vi "Begin.vi"(8 "error in":errorcluster) -> (0 "error out":errorcluster)   [LabVIEW 2017]
doc: "Called before other user functions, this VI is expected to open initial I/O refnums, load in file data, and do all program initialization. Notice that the <B>error out</B> terminal is simply used for data flow. Wiring it to other structures or subVIs ensures that this VI runs first."
uses:
  <vilib>/Rock Robotics/WPI/DriverStation/WPI_DriverStationRobotMode2.ctl
  <vilib>/Rock Robotics/WPI/Joystick/WPI_JoystickDeviceEnum.ctl
  <vilib>/Rock Robotics/WPI/SafetyOutput/WPI_SafetyOutputConfigMenu.ctl
  <vilib>/Rock Robotics/WPI/ThirdParty/Phoenix-LabVIEW/Motor Controller/Controls/CTRE_Phoenix_MotorControl_FeedbackDevice.ctl
  <vilib>/Rock Robotics/WPI/Solenoid/WPI_SolenoidChannel.ctl
  Robot Global Data.vi
  <vilib>/Rock Robotics/Network Tables/NT Write String Array.vi
  <vilib>/Rock Robotics/WPI/Utilities/WPI_GetSetVariantRefNum.vi
  <vilib>/Rock Robotics/WPI/RobotDrive/WPI_RobotDriveOpen4MotorWithExistingMotors.vi
  <vilib>/Rock Robotics/WPI/Solenoid/WPI_SolenoidOpenDouble.vi
  <vilib>/Rock Robotics/WPI/Solenoid/WPI_SolenoidOpenSingle.vi
  <vilib>/Rock Robotics/SystemInterfaces/spilib/spi_bus.ctl
  <vilib>/Rock Robotics/WPI/Gyro/WPI_GyroXRS450_SPI_Open.vi
  navx-mxp/labview/navX Library v2/navX Library v2.lvlib
  navx-mxp/labview/navX Library v2/IO/Open/Z900_navX_Open_I2C.vi
  <vilib>/Rock Robotics/SystemInterfaces/i2clib/i2c_bus.ctl
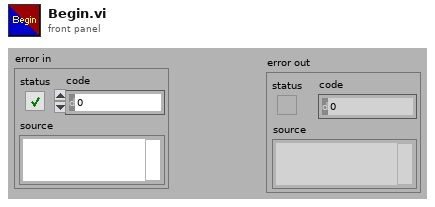
[diagram p1: front panel]
types:
  T1 = typedef "CTRE_Phoenix_MotorControl_FeedbackDevice.ctl" = i8
  T2 = typedef "WPI_JoystickDeviceEnum.ctl" = enum16{"USB 0", "USB 1", "USB 2", "USB 3", "USB 4", "USB 5"}
  T3 = typedef "WPI_SafetyOutputConfigMenu.ctl" = enum16{"Enable", "Disable"}
  T4 = typedef "WPI_DriverStationRobotMode2.ctl" = enum16{"Autonomous Disabled", "Autonomous Enabled", "Teleop Disabled", "Teleop Enabled", "Disconnected", "Finish", "Test Disabled", "Test Enabled", "Emergency Stopped"}
  T5 = typedef "WPI_MotorControlDeviceRef.ctl" = cluster{"DeviceStatus":errorcluster, "Type":T6, "PWM":cluster{"PWM Channel":T7, "DeadBand":T8}, "CAN":cluster{"Device Number":u8, "SetOutput VI Ref":variant, "GetOutput VI Ref":variant, "Enable VI Ref":variant, "Disable VI Ref":variant, "Data":variant}, "Invert":bool, "DIO PWM":cluster{"PWM \"Enable\" Channel":T7, "DIOChannel":T9, "PWM Rate":dbl}}
  T6 = typedef "WPI_MotorControlType.ctl" = enum16{"PWM", "CAN", "DIO PWM"}
  T7 = typedef "FPGA_DIOPWMChannel.ctl" = enum8{"PWM 0", "PWM 1", "PWM 2", "PWM 3", "PWM 4", "PWM 5", "PWM 6", "PWM 7", "PWM 8", "PWM 9", "PWM MXP 0", "PWM MXP 1", "PWM MXP 2", "PWM MXP 3", "PWM MXP 4", "PWM MXP 5", "PWM MXP 6", "PWM MXP 7", "PWM MXP 8", "PWM MXP 9", "Invalid"}
  T8 = typedef "WPI_PWMDeadband.ctl" = cluster{"Name":string, "maxPositivePwm":i32, "minPositivePwm":i32, "centerPwm":i32, "maxNegativePwm":i32, "minNegativePwm":i32, "angularRange":u16}
  T9 = typedef "FPGA_DIOChannel.ctl" = enum8{"DIO 0", "DIO 1", "DIO 2", "DIO 3", "DIO 4", "DIO 5", "DIO 6", "DIO 7", "DIO 8", "DIO 9", "DIO MXP 0", "DIO MXP 1", "DIO MXP 2", "DIO MXP 3", "DIO MXP 4", "DIO MXP 5", "DIO MXP 6", "DIO MXP 7", "DIO MXP 8", "DIO MXP 9", "DIO MXP 10", "DIO MXP 11", "DIO MXP 12", "DIO MXP 13", "DIO MXP 14", "DIO MXP 15", "SPI Port CS1", "SPI Port CS2", "SPI Port CS3", "SPI Port MISO", "SPI Port MOSI", "Invalid"}
  T10 = typedef "WPI_RobotDriveDevRef.ctl" = cluster{"DevStatus":errorcluster, "Motors[]":T5[], "Square Inputs":bool, "Max Output":dbl}
  T11 = typedef "i2c_bus.ctl" = enum16{"I2C On-Board", "I2C MXP", "Invalid"}
  T12 = typedef "navX Library v2.lvlib/Z900_navX_DeviceTypeDef.ctl" = cluster{"Interface":cluster{"Protocol":T13, "Update Rate (4Hz-100Hz)":u8, "navX Open TypeDef":variant}, "Notify Packet":refnum<notifier>, "Loop VI Refnum":refnum<vi>, "Ready to Close Occurrence Refnum":refnum<k4>}
  T13 = typedef "navX Library v2.lvlib/Z900_navX_ProtocolTypeDef.ctl" = enum16{"SERIAL", "I2C", "SPI"}
  T14 = typedef "spi_bus.ctl" = enum16{"SPI On-Board, CS0", "SPI On-Board, CS1", "SPI On-Board, CS2", "SPI On-Board, CS3", "SPI MXP", "Invalid"}
  T15 = typedef "WPI_GyroDevRef.ctl" = cluster{"DevStatus":errorcluster, "Analog Channel":T16, "Gain (VoltsPerDegree/Second)":dbl, "Gyro Type":enum16{"Analog", "XRS450"}, "Handle":i32, "SPI Bus":T14, "Device Found":bool, "Sample Rate":dbl, "Calibrate On Open":bool, "Offset":dbl}
  T16 = typedef "FPGA_AIChannel.ctl" = enum8{"AI 0", "AI 1", "AI 2", "AI 3", "AI MXP 0", "AI MXP 1", "AI MXP 2", "AI MXP 3", "Invalid"}
  T17 = typedef "WPI_SolenoidChannel.ctl" = enum8{"Solenoid 0", "Solenoid 1", "Solenoid 2", "Solenoid 3", "Solenoid 4", "Solenoid 5", "Solenoid 6", "Solenoid 7", "Invalid"}
  T18 = typedef "WPI_SolenoidDevRef.ctl" = cluster{"DevStatus":errorcluster, "Pneumatics Control Module":u8, "Forward Solenoid Channel":T17, "Reverse Solenoid Channel":T17}
  T19 = typedef "WPI_CompressorDevRef.ctl" = cluster{"DevStatus":errorcluster, "Pneumatics Control Module":u8}
  T20 = typedef "WPI_JoystickDevRef.ctl" = cluster{"Device":T2}
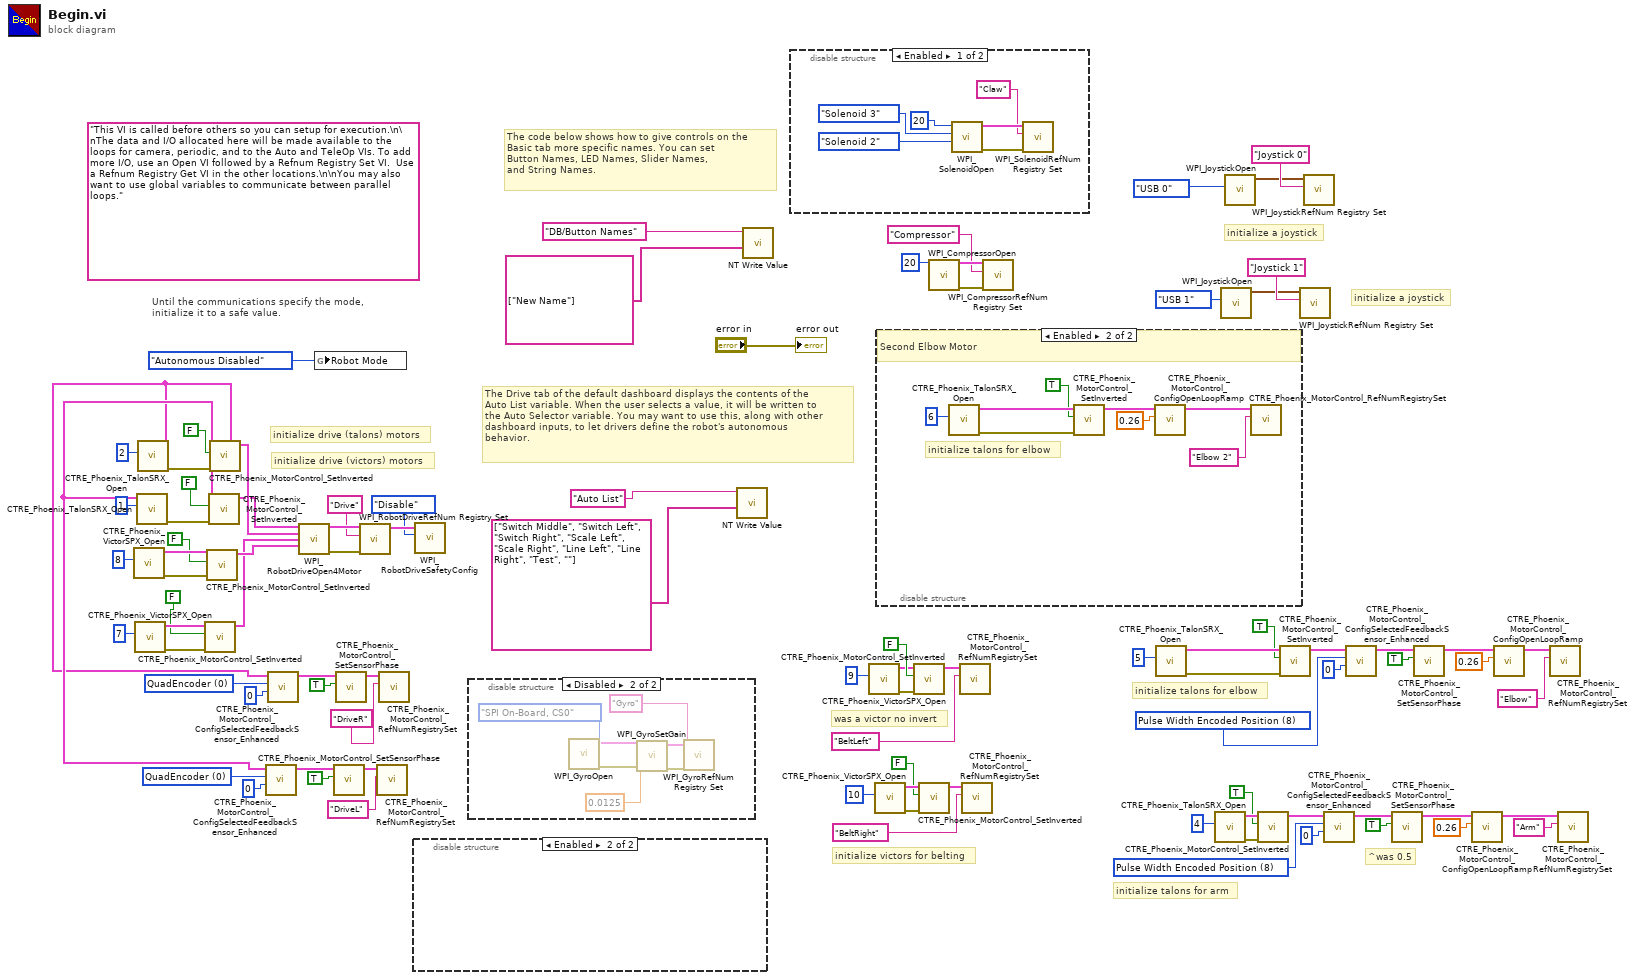
[diagram p0: block diagram]
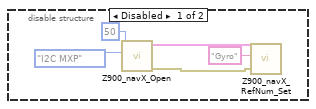
[diagram p2: hidden frame]
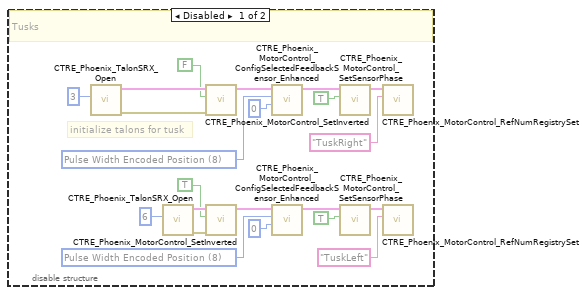
[diagram p4: hidden frame]
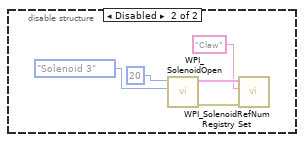
[diagram p5: hidden frame]
diagram:
  w18 = T1 8 items=["None"=-1, "QuadEncoder"=0, "Analog"=2, "Tachometer"=4, "Pulse Width Encoded Position"=8, "Sensor Sum (S0 + S1)"=9, "Sensor Difference (D0 - D1)"=10, "Remote Source 0"=11, "Remote Source 1"=12, "Software Emulated"=15] ("Feedback Device")
  w10 = T1 8 items=["None"=-1, "QuadEncoder"=0, "Analog"=2, "Tachometer"=4, "Pulse Width Encoded Position"=8, "Sensor Sum (S0 + S1)"=9, "Sensor Difference (D0 - D1)"=10, "Remote Source 0"=11, "Remote Source 1"=12, "Software Emulated"=15] ("Feedback Device")
  w56 = T1 0 items=["None"=-1, "QuadEncoder"=0, "Analog"=2, "Tachometer"=4, "Pulse Width Encoded Position"=8, "Sensor Sum (S0 + S1)"=9, "Sensor Difference (D0 - D1)"=10, "Remote Source 0"=11, "Remote Source 1"=12, "Software Emulated"=15] ("Feedback Device")
  w59 = T1 0 items=["None"=-1, "QuadEncoder"=0, "Analog"=2, "Tachometer"=4, "Pulse Width Encoded Position"=8, "Sensor Sum (S0 + S1)"=9, "Sensor Difference (D0 - D1)"=10, "Remote Source 0"=11, "Remote Source 1"=12, "Software Emulated"=15] ("Feedback Device")
  (unwired) "This VI is called before others so you can setup for execution.\n\nThe data and I/O allocated here will be made available to the loops for camera, periodic, and to the Auto and TeleOp VIs. To add more I/O, use an Open VI followed by a Refnum Registry Set VI.  Use a Refnum Registry Get VI in the other locations.\n\nYou may also want to use global variables to communicate between parallel loops."
  # "initialize a joystick"
  # "^was 0.5"
  # "was a victor no invert"
  # "initialize talons for elbow"
  # "initialize talons for arm"
  # "initialize victors for belting"
  # "initialize drive (victors) motors"
  # "initialize drive (talons) motors"
  # "The Drive tab of the default dashboard displays the contents of the\nAuto List variable. When the user selects a value, it will be written to\nthe Auto Selector variable. You may want to use this, along with other\ndashboard inputs, to let drivers define the robot's autonomous\nbehavior."
  # "The code below shows how to give controls on the\nBasic tab more specific names. You can set\nButton Names, LED Names, Slider Names,\nand String Names."
  # "initialize a joystick"
  # "Until the communications specify the mode,\ninitialize it to a safe value."
  n1 = call <vilib>:"CTRE_Phoenix_VictorSPX_Open.vi"("Device Number"=u8 8) -> ("error out"=w68:errorcluster, "CAN Talon SRX Ref"=w67:T5)  [unwired: 9 in]
  n2 = call <vilib>:"CTRE_Phoenix_VictorSPX_Open.vi"("Device Number"=u8 7) -> ("error out"=w65:errorcluster, "CAN Talon SRX Ref"=w66:T5)  [unwired: 9 in]
  n3 = call <vilib>:"CTRE_Phoenix_TalonSRX_Open.vi"("Device Number"=u8 1) -> ("error out"=w76:errorcluster, "CAN Talon SRX Ref"=w54:T5)  [unwired: 9 in]
  n4 = call <vilib>:"CTRE_Phoenix_TalonSRX_Open.vi"("Device Number"=u8 2) -> ("error out"=w75:errorcluster, "CAN Talon SRX Ref"=w47:T5)  [unwired: 9 in]
  n5 = call <vilib>:"CTRE_Phoenix_MotorControl_SetInverted.vi"("error in (no error)"=w65, "Invert?"=FALSE, "PhoenixMotorControlDevRef"=w66) -> ("PhoenixMotorControlDevRef"=w21:T5)  [unwired: 7 in, 1 out]
  n6 = call <vilib>:"CTRE_Phoenix_MotorControl_SetInverted.vi"("error in (no error)"=w68, "Invert?"=FALSE, "PhoenixMotorControlDevRef"=w67) -> ("PhoenixMotorControlDevRef"=w22:T5)  [unwired: 7 in, 1 out]
  n7 = call <vilib>:"CTRE_Phoenix_MotorControl_SetInverted.vi"("error in (no error)"=w76, "Invert?"=FALSE, "PhoenixMotorControlDevRef"=w54) -> ("PhoenixMotorControlDevRef"=w23:T5)  [unwired: 7 in, 1 out]
  n8 = call <vilib>:"CTRE_Phoenix_MotorControl_SetInverted.vi"("error in (no error)"=w75, "Invert?"=FALSE, "PhoenixMotorControlDevRef"=w47) -> ("PhoenixMotorControlDevRef"=w24:T5)  [unwired: 7 in, 1 out]
  n9 = call <vilib>:"CTRE_Phoenix_MotorControl_ConfigSelectedFeedbackSensor_Enhanced.vi"("pidLoopIdx"=0, "Feedback Device"=w56, "PhoenixMotorControlDevRef"=w54) -> ("PhoenixMotorControlDevRef"=w50:T5)  [unwired: 7 in, 1 out]
  n10 = call <vilib>:"CTRE_Phoenix_MotorControl_ConfigSelectedFeedbackSensor_Enhanced.vi"("pidLoopIdx"=0, "Feedback Device"=w59, "PhoenixMotorControlDevRef"=w47) -> ("PhoenixMotorControlDevRef"=w53:T5)  [unwired: 7 in, 1 out]
  n11 = call-poly <vilib>:"WPI_RobotDriveOpen4Motor.vi"("Rear Left Motor Dev Ref"=w23, "Rear Right Motor Dev Ref"=w24, "Front Left Motor Dev Ref"=w21, "Front Right Motor Dev Ref"=w22) -> ("RobotDriveDevRef"=w79:T10, "error out"=w78:errorcluster)  [unwired: 10 in]
  n12 = global write "Robot Global Data.vi" "Robot Mode"(WPI_DriverStationRobotMode2."Autonomous Disabled" ("Robot Mode")) -> ()
  n13 = call <vilib>:"CTRE_Phoenix_MotorControl_SetSensorPhase.vi"("PhaseSensor"=TRUE, "PhoenixMotorControlDevRef"=w50) -> ("PhoenixMotorControlDevRef"=w49:T5)  [unwired: 8 in, 1 out]
  n14 = call <vilib>:"CTRE_Phoenix_MotorControl_SetSensorPhase.vi"("PhaseSensor"=TRUE, "PhoenixMotorControlDevRef"=w53) -> ("PhoenixMotorControlDevRef"=w52:T5)  [unwired: 8 in, 1 out]
  n15 = call <vilib>:"WPI_RobotDriveRefNum Registry Set.vi"("error in (no error)"=w78, "refnum name"="Drive", "RobotDriveDevRef"=w79) -> ("RobotDriveDevRef"=w80:T10)  [unwired: 7 in, 1 out]
  n16 = call <vilib>:"CTRE_Phoenix_MotorControl_RefNumRegistrySet.vi"("refnum name"="DriveL", "PhoenixMotorControlDevRef"=w49) -> ()  [unwired: 8 in, 2 out]
  n17 = call <vilib>:"CTRE_Phoenix_MotorControl_RefNumRegistrySet.vi"("refnum name"="DriveR", "PhoenixMotorControlDevRef"=w52) -> ()  [unwired: 8 in, 2 out]
  n18 = disable-structure shown="Enabled" {
    frame Disabled {
      n19 = call-poly "Z900_navX_Open.vi"("I2C Bus"=i2c_bus."I2C MXP", "Update Rate (4Hz-60Hz)"=50) -> ("error out"=w93:errorcluster, "navX Device"=w95:T12)  [unwired: 8 in]
      n20 = call "Z900_navX_RefNum_Set.vi"("error in (no error)"=w93, "refnum name"="Gyro", "navX Device"=w95) -> ()  [unwired: 7 in, 2 out]
    }
    frame Enabled {
    }
  }
  n21 = call <vilib>:"WPI_RobotDriveSafetyConfig.vi"("mode"=WPI_SafetyOutputConfigMenu."Disable", "RobotDriveDevRef"=w80) -> ()  [unwired: 8 in, 2 out]
  n22 = disable-structure shown="Disabled" {
    frame Enabled {
      # "U DISABLED BOI"
    }
    frame Disabled {
      n23 = call-poly <vilib>:"WPI_GyroOpen.vi"("SPI Bus"=spi_bus."SPI On-Board, CS0") -> ("error out"=w98:errorcluster, "GyroDevRef"=w101:T15)  [unwired: 8 in, 1 out]
      n24 = call <vilib>:"WPI_GyroSetGain.vi"("error in (no error)"=w98, "Gain (VoltsPerDegree/Second)"=0.0125, "GyroDevRef"=w101) -> ("error out"=w97:errorcluster, "GyroDevRef"=w100:T15)  [unwired: 7 in]
      n25 = call <vilib>:"WPI_GyroRefNum Registry Set.vi"("error in (no error)"=w97, "refnum name"="Gyro", "GyroDevRef"=w100) -> ()  [unwired: 7 in, 2 out]
    }
  }
  n26 = call-poly <vilib>:"NT Write Value.vi"("String Array"=string[] ["Switch Middle", "Switch Left", "Switch Right", "Scale Left", "Scale Right", "Line Left", "Line Right", "Test", ""], "Name"="Auto List") -> ()  [unwired: 9 in, 1 out]
  n27 = call-poly <vilib>:"NT Write Value.vi"("String Array"=string[] ["New Name"], "Name"="DB/Button Names") -> ()  [unwired: 9 in, 1 out]
  n28 = disable-structure shown="Enabled" {
    frame Enabled {
      n29 = call-poly <vilib>:"WPI_SolenoidOpen.vi"("Reverse Solenoid Channel"=WPI_SolenoidChannel."Solenoid 2", "Forward Solenoid Channel"=WPI_SolenoidChannel."Solenoid 3", "Pneumatics Control Module (0)"=u8 20) -> ("error out"=w108:errorcluster, "SolenoidDevRef"=w109:T18)  [unwired: 7 in]
      n30 = call <vilib>:"WPI_SolenoidRefNum Registry Set.vi"("error in (no error)"=w108, "refnum name"="Claw", "SolenoidDevRef"=w109) -> ()  [unwired: 7 in, 2 out]
    }
    frame Disabled {
      n31 = call-poly <vilib>:"WPI_SolenoidOpen.vi"("Solenoid Channel"=WPI_SolenoidChannel."Solenoid 3" ("Forward Solenoid Channel"), "Pneumatics Control Module (0)"=u8 20) -> ("error out"=w113:errorcluster, "SolenoidDevRef"=w114:T18)  [unwired: 8 in]
      n32 = call <vilib>:"WPI_SolenoidRefNum Registry Set.vi"("error in (no error)"=w113, "refnum name"="Claw", "SolenoidDevRef"=w114) -> ()  [unwired: 7 in, 2 out]
    }
  }
  n33 = call <vilib>:"CTRE_Phoenix_VictorSPX_Open.vi"("Device Number"=u8 9) -> ("error out"=w3:errorcluster, "CAN Talon SRX Ref"=w4:T5)  [unwired: 9 in]
  n34 = call <vilib>:"CTRE_Phoenix_VictorSPX_Open.vi"("Device Number"=u8 10) -> ("error out"=w42:errorcluster, "CAN Talon SRX Ref"=w45:T5)  [unwired: 9 in]
  n35 = disable-structure shown="Enabled" {
    frame Disabled {
      w125 = T1 8 items=["None"=-1, "QuadEncoder"=0, "Analog"=2, "Tachometer"=4, "Pulse Width Encoded Position"=8, "Sensor Sum (S0 + S1)"=9, "Sensor Difference (D0 - D1)"=10, "Remote Source 0"=11, "Remote Source 1"=12, "Software Emulated"=15] ("Feedback Device")
      w117 = T1 8 items=["None"=-1, "QuadEncoder"=0, "Analog"=2, "Tachometer"=4, "Pulse Width Encoded Position"=8, "Sensor Sum (S0 + S1)"=9, "Sensor Difference (D0 - D1)"=10, "Remote Source 0"=11, "Remote Source 1"=12, "Software Emulated"=15] ("Feedback Device")
      # "initialize talons for tusk"
      # "Tusks"
      n36 = call <vilib>:"CTRE_Phoenix_TalonSRX_Open.vi"("Device Number"=u8 3) -> ("error out"=w129:errorcluster, "CAN Talon SRX Ref"=w133:T5)  [unwired: 9 in]
      n37 = call <vilib>:"CTRE_Phoenix_TalonSRX_Open.vi"("Device Number"=u8 6) -> ("error out"=w130:errorcluster, "CAN Talon SRX Ref"=w134:T5)  [unwired: 9 in]
      n38 = call <vilib>:"CTRE_Phoenix_MotorControl_SetInverted.vi"("error in (no error)"=w129, "Invert?"=FALSE, "PhoenixMotorControlDevRef"=w133) -> ("PhoenixMotorControlDevRef"=w118:T5)  [unwired: 7 in, 1 out]
      n39 = call <vilib>:"CTRE_Phoenix_MotorControl_SetInverted.vi"("error in (no error)"=w130, "Invert?"=TRUE, "PhoenixMotorControlDevRef"=w134) -> ("PhoenixMotorControlDevRef"=w119:T5)  [unwired: 7 in, 1 out]
      n40 = call <vilib>:"CTRE_Phoenix_MotorControl_ConfigSelectedFeedbackSensor_Enhanced.vi"("pidLoopIdx"=0, "Feedback Device"=w125, "PhoenixMotorControlDevRef"=w118) -> ("PhoenixMotorControlDevRef"=w123:T5)  [unwired: 7 in, 1 out]
      n41 = call <vilib>:"CTRE_Phoenix_MotorControl_ConfigSelectedFeedbackSensor_Enhanced.vi"("pidLoopIdx"=0, "Feedback Device"=w117, "PhoenixMotorControlDevRef"=w119) -> ("PhoenixMotorControlDevRef"=w121:T5)  [unwired: 7 in, 1 out]
      n42 = call <vilib>:"CTRE_Phoenix_MotorControl_SetSensorPhase.vi"("PhaseSensor"=TRUE, "PhoenixMotorControlDevRef"=w123) -> ("PhoenixMotorControlDevRef"=w116:T5)  [unwired: 8 in, 1 out]
      n43 = call <vilib>:"CTRE_Phoenix_MotorControl_SetSensorPhase.vi"("PhaseSensor"=TRUE, "PhoenixMotorControlDevRef"=w121) -> ("PhoenixMotorControlDevRef"=w115:T5)  [unwired: 8 in, 1 out]
      n44 = call <vilib>:"CTRE_Phoenix_MotorControl_RefNumRegistrySet.vi"("refnum name"="TuskRight", "PhoenixMotorControlDevRef"=w116) -> ()  [unwired: 8 in, 2 out]
      n45 = call <vilib>:"CTRE_Phoenix_MotorControl_RefNumRegistrySet.vi"("refnum name"="TuskLeft", "PhoenixMotorControlDevRef"=w115) -> ()  [unwired: 8 in, 2 out]
    }
    frame Enabled {
      # "initialize talons for elbow"
      # "Second Elbow Motor"
      n46 = call <vilib>:"CTRE_Phoenix_TalonSRX_Open.vi"("Device Number"=u8 6) -> ("error out"=w141:errorcluster, "CAN Talon SRX Ref"=w143:T5)  [unwired: 9 in]
      n47 = call <vilib>:"CTRE_Phoenix_MotorControl_SetInverted.vi"("error in (no error)"=w141, "Invert?"=TRUE, "PhoenixMotorControlDevRef"=w143) -> ("PhoenixMotorControlDevRef"=w137:T5)  [unwired: 7 in, 1 out]
      n48 = call <vilib>:"CTRE_Phoenix_MotorControl_ConfigOpenLoopRamp.vi"("secondsFromNeutralToFull"=0.26, "PhoenixMotorControlDevRef"=w137) -> ("PhoenixMotorControlDevRef"=w138:T5)  [unwired: 8 in, 1 out]
      n49 = call <vilib>:"CTRE_Phoenix_MotorControl_RefNumRegistrySet.vi"("refnum name"="Elbow 2", "PhoenixMotorControlDevRef"=w138) -> ()  [unwired: 8 in, 2 out]
    }
  }
  n50 = call <vilib>:"CTRE_Phoenix_MotorControl_SetInverted.vi"("error in (no error)"=w3, "Invert?"=FALSE, "PhoenixMotorControlDevRef"=w4) -> ("PhoenixMotorControlDevRef"=w41:T5)  [unwired: 7 in, 1 out]
  n51 = call <vilib>:"CTRE_Phoenix_MotorControl_SetInverted.vi"("error in (no error)"=w42, "Invert?"=FALSE, "PhoenixMotorControlDevRef"=w45) -> ("PhoenixMotorControlDevRef"=w39:T5)  [unwired: 7 in, 1 out]
  n52 = call <vilib>:"WPI_CompressorOpen.vi"("Pneumatics Control Module (0)"=u8 20) -> ("CompressorDevRef"=w72:T19, "error out"=w71:errorcluster)  [unwired: 13 in]
  n53 = call <vilib>:"CTRE_Phoenix_MotorControl_RefNumRegistrySet.vi"("refnum name"="BeltLeft", "PhoenixMotorControlDevRef"=w41) -> ()  [unwired: 8 in, 2 out]
  n54 = call <vilib>:"CTRE_Phoenix_MotorControl_RefNumRegistrySet.vi"("refnum name"="BeltRight", "PhoenixMotorControlDevRef"=w39) -> ()  [unwired: 8 in, 2 out]
  n55 = call <vilib>:"WPI_CompressorRefNum Registry Set.vi"("error in (no error)"=w71, "refnum name"="Compressor", "CompressorDevRef"=w72) -> ()  [unwired: 7 in, 2 out]
  n56 = call <vilib>:"CTRE_Phoenix_TalonSRX_Open.vi"("Device Number"=u8 5) -> ("error out"=w28:errorcluster, "CAN Talon SRX Ref"=w32:T5)  [unwired: 9 in]
  n57 = call <vilib>:"CTRE_Phoenix_TalonSRX_Open.vi"("Device Number"=u8 4) -> ("error out"=w27:errorcluster, "CAN Talon SRX Ref"=w31:T5)  [unwired: 9 in]
  n58 = call <vilib>:"WPI_JoystickOpen.vi"("JoystickDevice"=WPI_JoystickDeviceEnum."USB 1") -> ("JoystickDevRef"=w36:T20)  [unwired: 10 in]
  n59 = call <vilib>:"WPI_JoystickOpen.vi"("JoystickDevice"=WPI_JoystickDeviceEnum."USB 0") -> ("JoystickDevRef"=w89:T20)  [unwired: 10 in]
  n60 = call <vilib>:"CTRE_Phoenix_MotorControl_SetInverted.vi"("error in (no error)"=w27, "Invert?"=TRUE, "PhoenixMotorControlDevRef"=w31) -> ("PhoenixMotorControlDevRef"=w12:T5)  [unwired: 7 in, 1 out]
  n61 = call <vilib>:"CTRE_Phoenix_MotorControl_SetInverted.vi"("error in (no error)"=w28, "Invert?"=TRUE, "PhoenixMotorControlDevRef"=w32) -> ("PhoenixMotorControlDevRef"=w14:T5)  [unwired: 7 in, 1 out]
  n62 = call <vilib>:"WPI_JoystickRefNum Registry Set.vi"("refnum name"="Joystick 1", "JoystickDevRef"=w36) -> ()  [unwired: 8 in, 2 out]
  n63 = call <vilib>:"WPI_JoystickRefNum Registry Set.vi"("refnum name"="Joystick 0", "JoystickDevRef"=w89) -> ()  [unwired: 8 in, 2 out]
  n64 = call <vilib>:"CTRE_Phoenix_MotorControl_ConfigSelectedFeedbackSensor_Enhanced.vi"("pidLoopIdx"=0, "Feedback Device"=w18, "PhoenixMotorControlDevRef"=w12) -> ("PhoenixMotorControlDevRef"=w16:T5)  [unwired: 7 in, 1 out]
  n65 = call <vilib>:"CTRE_Phoenix_MotorControl_ConfigSelectedFeedbackSensor_Enhanced.vi"("pidLoopIdx"=0, "Feedback Device"=w10, "PhoenixMotorControlDevRef"=w14) -> ("PhoenixMotorControlDevRef"=w13:T5)  [unwired: 7 in, 1 out]
  n66 = call <vilib>:"CTRE_Phoenix_MotorControl_SetSensorPhase.vi"("PhaseSensor"=TRUE, "PhoenixMotorControlDevRef"=w16) -> ("PhoenixMotorControlDevRef"=w8:T5)  [unwired: 8 in, 1 out]
  n67 = call <vilib>:"CTRE_Phoenix_MotorControl_SetSensorPhase.vi"("PhaseSensor"=TRUE, "PhoenixMotorControlDevRef"=w13) -> ("PhoenixMotorControlDevRef"=w9:T5)  [unwired: 8 in, 1 out]
  n68 = call <vilib>:"CTRE_Phoenix_MotorControl_ConfigOpenLoopRamp.vi"("secondsFromNeutralToFull"=0.26, "PhoenixMotorControlDevRef"=w8) -> ("PhoenixMotorControlDevRef"=w2:T5)  [unwired: 8 in, 1 out]
  n69 = call <vilib>:"CTRE_Phoenix_MotorControl_ConfigOpenLoopRamp.vi"("secondsFromNeutralToFull"=0.26, "PhoenixMotorControlDevRef"=w9) -> ("PhoenixMotorControlDevRef"=w1:T5)  [unwired: 8 in, 1 out]
  n70 = call <vilib>:"CTRE_Phoenix_MotorControl_RefNumRegistrySet.vi"("refnum name"="Elbow", "PhoenixMotorControlDevRef"=w1) -> ()  [unwired: 8 in, 2 out]
  n71 = call <vilib>:"CTRE_Phoenix_MotorControl_RefNumRegistrySet.vi"("refnum name"="Arm", "PhoenixMotorControlDevRef"=w2) -> ()  [unwired: 8 in, 2 out]
  "error out" <- "error in"
